vi "WorkorderHandler_getStatus.vi"(0 "reference":T1, 5 "error in (no error)":errorcluster) -> (12 "object name":string, 14 "duplicate reference":T1, 15 "methods pending lock":i32, 17 "object locked":bool, 19 "error out":errorcluster)   [LabVIEW 2011]
doc: "Returns the current state of the dqGOOP object"
uses:
  DataStructures/WorkorderHandler_ObjectReference.ctl
  DataStructures/WorkorderHandler_ObjectData.ctl
panel:
  in  "queue (default)":refnum<queue>
  # "Copyright (C) 2004 DataAct Incorporated"
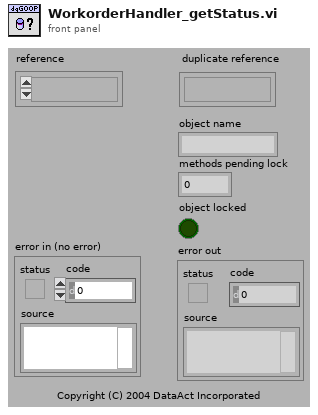
[diagram p1: front panel]
types:
  T1 = typedef "WorkorderHandler_ObjectReference.ctl" = refnum<k1>
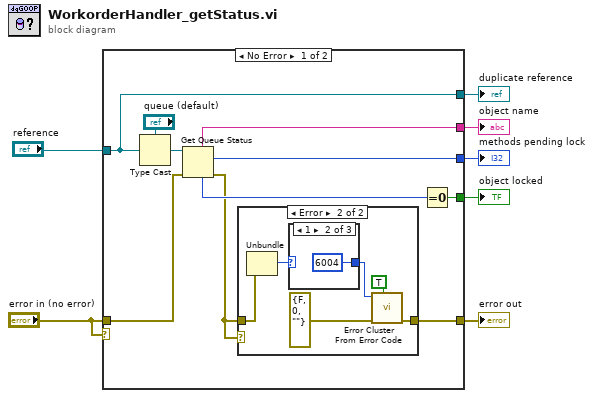
[diagram p0: block diagram]
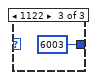
[diagram p4: hidden frame]
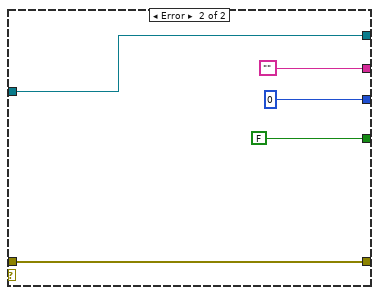
[diagram p5: hidden frame]
diagram:
  n1 = case shown="No Error" "error in (no error)" {
    tunnel: [w8 w28] -> w7
    tunnel: [w15 FALSE] -> w3
    tunnel: "reference" -> [w10 w31]
    tunnel: [w10 w31] -> w5
    tunnel: [w17 ""] -> w4
    tunnel: [w14 0] -> w2
    tunnel: "error in (no error)" -> [w13 w28]
    frame No Error {
      n2 = Type Cast(type="queue (default)", x=w10) -> (*(type *) &x=w11:refnum<queue>)
      n3 = Get Queue Status(queue=w11, error in (no error)=w13) -> (queue name=w17:string, # pending remove=w14:i32, error out=w9:errorcluster, # elements in queue=w16:i32)  [unwired: 1 in, 4 out]
      n4 = case shown="Error" w9 {
        tunnel: [w18 w19] -> w8
        tunnel: w9 -> [w18 w24]
        frame No Error {
        }
        frame Error {
          n5 = Unbundle(w24) -> ("code"=w23:i32)  [unwired: 2 out]
          n6 = case shown="1" w23 {
            selector: w23 -> [w25 _ _]
            tunnel: [w25 6004 ("code") 6003 ("code")] -> w21
            frame Default {
            }
            frame 1 {
            }
            frame 1122 {
            }
          }
          n7 = call <vilib>:"Error Cluster From Error Code.vi"("show call chain? (False)"=TRUE, "error in (no error)"=errorcluster {"status"=FALSE, "code"=0, "source"=""} ("error out"), "error code (0)"=w21) -> ("error out"=w19:errorcluster)  [unwired: 6 out]
        }
      }
      n8 = Equal To 0?(x=w16) -> (x = 0?=w15:bool)
    }
    frame Error {
    }
  }
  "error out" <- w7
  "object locked" <- w3
  "duplicate reference" <- w5
  "object name" <- w4
  "methods pending lock" <- w2
